vi "SEK2020c1VI3AprenderOrdemCores.vi"(0 "ordem das cores 2":T1, 8 "Parâmetros 2":T3={"Azul Max EV3 Cor"=17, "Azul Min EV3 Cor"=0, "Verde Max EV3 Cor"=6, "Verde Min EV3 Cor"=0, "Vermelho Max Ev3 Cor"=0, "Vermelho Min EV3 Cor"=0, "Chão EV3 Cor"=0.0, "Branco Max EV3 Cor"=0.0, "Branco Min EV3 Cor"=0.0, "Preto Max EV3 Cor"=0.0, "Preto Min EV3 Cor"=0.0, "Distância Tubulação"=0.0, "Distância Frontal"=0.0, "Amarelo Max EV3 Cor"=0.0, "Amarelo Min EV3 Cor"=0.0, "Distância Lateral"=0.0, "90°"=0.0, "180°"=0.0, "Seguidor de Linha"=0.0}, 11 "NXT/EV3 2":T2) -> (3 "NXT/EV3 13":T2)   [LabVIEW 2016]
uses:
  <vilib>/NXT/Subs/LVHSConnector.ctl
  <vilib>/NXT/LegoClasses/BrickReference/BrickReference.lvclass
  <vilib>/NXT/Block Support/NXT_InputPort.ctl
  <vilib>/NXT/Dual Mode Library/Sensors/EV3_Color_Reflect.vi
  <vilib>/NXT/NXTIO Xnodes/AddressXNode/NXTIOAddress.xnode
panel:
  out "primeira cor":dbl format="%#_13g"
  out "y3":dbl format="%#_13g"
  out "terceira cor":dbl format="%#_13g"
  out "y1":dbl format="%#_13g"
  out "y2":dbl format="%#_13g"
  out "segunda cor":dbl format="%#_13g"
  # "Sensor EV3 Cor"
  # "Sensor Ultrassônico"
  # "Sensor Giroscópio"
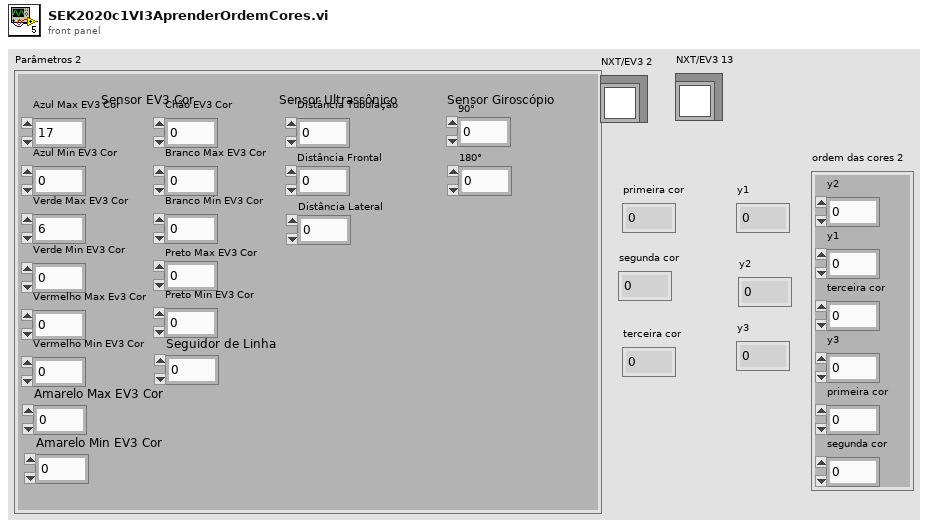
[diagram p1: front panel]
types:
  T1 = cluster{"y2":dbl, "y1":dbl, "terceira cor":dbl, "y3":dbl, "primeira cor":dbl, "segunda cor":dbl}
  T2 = typedef "LVHSConnector.ctl" = refnum<class "BrickReference.lvclass">
  T3 = cluster{"Azul Max EV3 Cor":i32, "Azul Min EV3 Cor":i32, "Verde Max EV3 Cor":i32, "Verde Min EV3 Cor":i32, "Vermelho Max Ev3 Cor":i32, "Vermelho Min EV3 Cor":i32, "Chão EV3 Cor":sgl, "Branco Max EV3 Cor":sgl, "Branco Min EV3 Cor":sgl, "Preto Max EV3 Cor":sgl, "Preto Min EV3 Cor":sgl, "Distância Tubulação":sgl, "Distância Frontal":sgl, "Amarelo Max EV3 Cor":dbl, "Amarelo Min EV3 Cor":dbl, "Distância Lateral":sgl, "90°":sgl, "180°":sgl, "Seguidor de Linha":dbl}
  T4 = typedef "NXT_InputPort.ctl" = u32
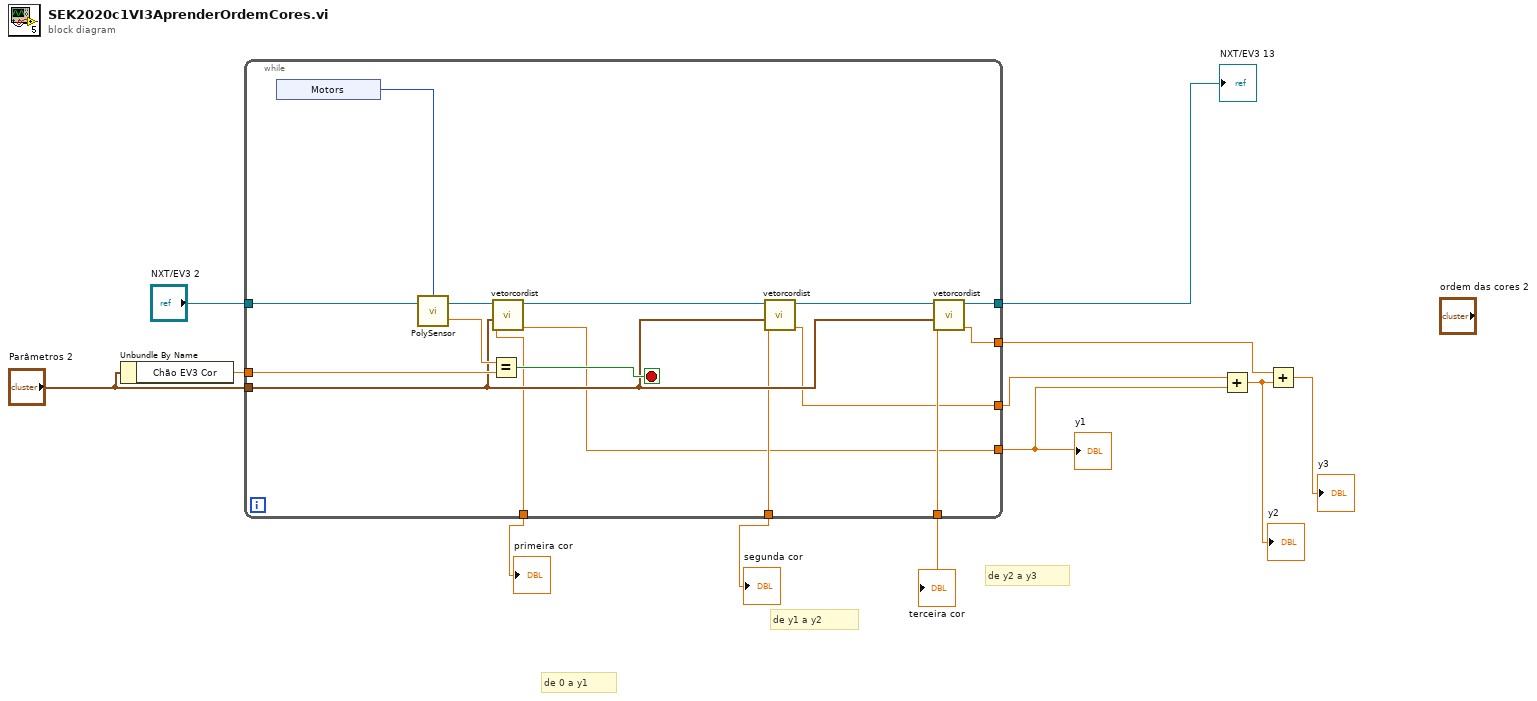
[diagram p0: block diagram]
diagram:
  # "de y2 a y3"
  # "de y1 a y2"
  # "de 0 a y1"
  n1 = Unbundle By Name("Parâmetros 2") -> ("Chão EV3 Cor"=w12:sgl)
  n2 = while {
    tunnel: w12 -> [w28]
    tunnel: "NXT/EV3 2" -> [w27]
    tunnel: [w21] -> w10
    tunnel: "Parâmetros 2" -> [w19]
    tunnel: [w18] -> w6
    tunnel: [w17] -> w5
    tunnel: [w16] -> w4
    tunnel: [w15] -> w3
    tunnel: [w14] -> w2
    tunnel: [w13] -> w1
    stop <- w20 stop-if-true
    n3 = xnode "Motors"() -> ("Sensor"=w25:T4)
    n4 = call-poly <vilib>:"PolySensor.vi"("NXT/EV3"=w27, "Port (Port 1)"=w25) -> ("Scaled Value"=w26:sgl, "NXT/EV3"=w24:T2)  [unwired: 1 in]
    n5 = Equal?(x=w26, y=w28) -> (x = y?=w20:bool)
    n6 = call "vetorcordist.vi"("Parâmetros 2"=w19, "NXT/EV3 2"=w24) -> ("dist perc"=w15:dbl, "NXT/EV3 13"=w23:T2, "cod cor"=w18:dbl)  [unwired: 7 in]
    n7 = call "vetorcordist.vi"("Parâmetros 2"=w19, "NXT/EV3 2"=w23) -> ("dist perc"=w14:dbl, "NXT/EV3 13"=w22:T2, "cod cor"=w17:dbl)  [unwired: 7 in]
    n8 = call "vetorcordist.vi"("Parâmetros 2"=w19, "NXT/EV3 2"=w22) -> ("dist perc"=w13:dbl, "NXT/EV3 13"=w21:T2, "cod cor"=w16:dbl)  [unwired: 7 in]
  }
  "NXT/EV3 13" <- w10
  "segunda cor" <- w5
  "y1" <- w3
  "terceira cor" <- w4
  "primeira cor" <- w6
  n9 = Add(x=w2, y=w3) -> (x+y=w8:dbl)
  "y2" <- w8
  n10 = Add(x=w1, y=w8) -> (x+y=→"y3":dbl)
